vi "get_current_valve.vi"(8 "error in (no error)":errorcluster, 10 "total reactors":u32, 11 "VISA Refnum in":refnum<visa-resource-name>) -> (0 "error out":errorcluster, 2 "LAST VALVE":i32, 3 "VISA Refnum out":refnum<visa-resource-name>)   [LabVIEW 2013]
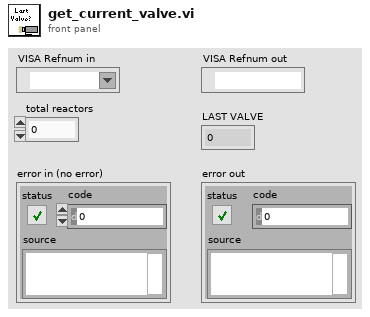
[diagram p1: front panel]
types:
  T1 = enum16{"Move to Home", "Set Positions", "Set Actuator Mode", "OTHER", "Set Direction", "CW Move", "CCW Move"}
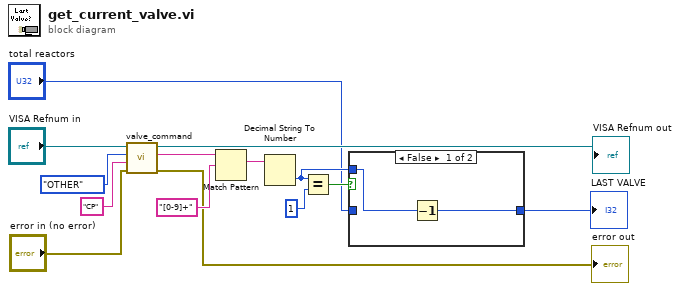
[diagram p0: block diagram]
diagram:
  n1 = call "valve_command.vi"("Error IN"="error in (no error)", "Command option"="CP", "COMMANDS"=T1."OTHER", "VALVE PORT IN"="VISA Refnum in") -> ("Error OUT"=→"error out":errorcluster, "read buffer"=w7:string, "VALVE PORT OUT"=→"VISA Refnum out":refnum<visa-resource-name>)  [unwired: 5 in]
  n2 = Match Pattern(string=w7, regular expression="[0-9]+") -> (match substring=w14:string)  [unwired: 1 in, 3 out]
  n3 = Decimal String To Number(string=w14) -> (number=w3:i32)  [unwired: 2 in, 1 out]
  n4 = Equal?(x=w3, y=1) -> (x = y?=w5:bool)
  n5 = case shown="False" w5 {
    tunnel: w3 -> [w16 _]
    tunnel: "total reactors" -> [_ w17]
    tunnel: [w15 w17] -> w1
    frame False {
      n6 = Decrement(x=w16) -> (x-1=w15:i32)
    }
    frame True {
    }
  }
  "LAST VALVE" <- w1
